vi "CalculateInputString_v2.vi"(1 "Rad":bool, 2 "InputString":string="1 + 2 * 4") -> (0 "result":dbl format="%.2f")   [LabVIEW 2016]
uses:
  <vilib>/gmath/NI_Gmath.lvlib
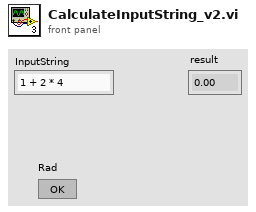
[diagram p1: front panel]
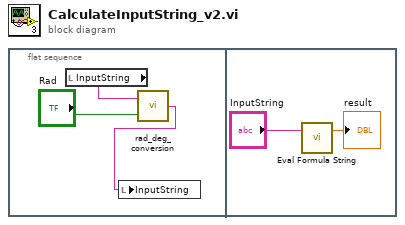
[diagram p0: block diagram]
diagram:
  n1 = flat-sequence {
    frame #0 {
      n2 = local read "InputString"() -> (w2:string)
      n3 = call "rad_deg_conversion.vi"("Rad"="Rad", "InputString"=w2) -> ("result"=w1:string)
      n4 = local write "InputString"(w1) -> ()
    }
    frame #1 {
      n5 = call <vilib>:"Eval Formula String.vi"("formula"="InputString") -> ("y value"=→"result":dbl)  [unwired: 1 in, 1 out]
    }
  }
